vi "Serial_Terminal.vi"() -> ()   [LabVIEW 2009]
uses:
  <vilib>/Instr/_visa.llb/VISA Configure Serial Port (Instr).vi
panel:
  in  "baud rate (9600)":u32=38400
  in  "Send Style":u16(ring) items=["Slash Codes"=1, "HEX"=3, "ASCII"=0]
  in  "Send":bool
  in  "Input":string
  in  "Selection Style":u16(ring)=3 items=["Slash Codes"=1, "HEX"=3, "ASCII"=0]
  out "concatenated string 2":string
  in  "Display Style":u16(ring) items=["Slash Codes"=1, "HEX"=3, "ASCII"=0]
  in  "reset":bool
  in  "clear":bool
  in  "start/stop":bool=TRUE
  in  "VISA resource name":refnum<visa-resource-name>
  out "concatenated string":string
  in  "stop":bool
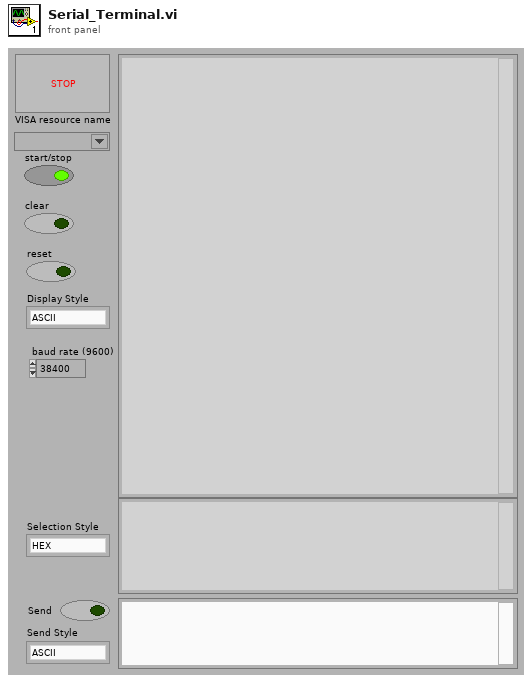
[diagram p1: front panel]
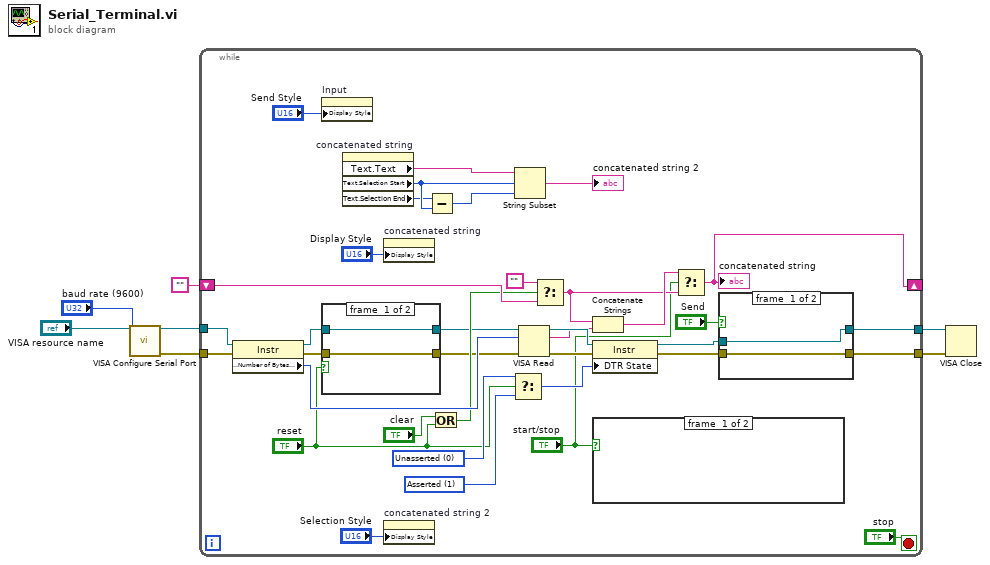
[diagram p0: block diagram]
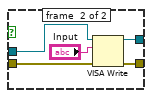
[diagram p2: hidden frame]
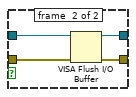
[diagram p3: hidden frame]
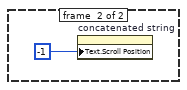
[diagram p4: hidden frame]
diagram:
  n1 = call-poly "VISA Configure Serial Port"("VISA resource name"="VISA resource name", "baud rate (9600)"="baud rate (9600)") -> ("VISA resource name out"=w5:refnum<visa-resource-name>, "error out"=w6:errorcluster)  [unwired: 12 in]
  n2 = while {
    shift-right: [w39] -> _
    shift-left: "" -> [w37]
    tunnel: w5 -> [w9]
    tunnel: w6 -> [w8]
    tunnel: [w11] -> w4
    tunnel: [w10] -> w3
    stop <- "stop" stop-if-true
    w34 = i16 1 items=["Unknown"=-1, "Unasserted"=0, "Asserted"=1] ("Serial Settings:Modem Line Settings:Line DTR State")
    w35 = i16 0 items=["Unknown"=-1, "Unasserted"=0, "Asserted"=1] ("Serial Settings:Modem Line Settings:Line DTR State")
    n3 = property class="Instr"(reference=w9, error in=w8) -> (reference out=w25:refnum<visa-resource-name>, error out=w24:errorcluster, "Serial Settings:Number of Bytes at Serial Port"=w42:u32)
    n4 = property on="Input" class="Str"("Display Style"="Send Style") -> ()  [unwired: 2 in, 2 out]
    n5 = case shown="False" "reset" {
      tunnel: w25 -> [w52 w56]
      tunnel: [w52 w55] -> w22
      tunnel: w24 -> [w51 w54]
      tunnel: [w51 w53] -> w23
      frame #0 {
      }
      frame #1 {
        n6 = VISA Flush I/O Buffer(VISA resource name=w56, error in (no error)=w54) -> (VISA resource name out=w55:refnum<visa-resource-name>, error out=w53:errorcluster)  [unwired: 1 in]
      }
    }
    n7 = property on="concatenated string" class="Str"() -> ("Text.Text"=w21:string, "Text.Selection Start"=w20:u32, "Text.Selection End"=w19:u32)  [unwired: 2 in, 2 out]
    n8 = property on="concatenated string" class="Str"("Display Style"="Display Style") -> ()  [unwired: 2 in, 2 out]
    n9 = property on="concatenated string 2" class="Str"("Display Style"="Selection Style") -> ()  [unwired: 2 in, 2 out]
    n10 = Subtract(x=w19, y=w20) -> (x-y=w18:u32)
    n11 = Or(x="clear", y="reset") -> (x .or. y?=w27:bool)
    n12 = Select(t=w35, s="reset", f=w34) -> (s? t:f=w33:i16)
    n13 = String Subset(string=w21, offset (0)=w20, length (rest)=w18) -> (substring=→"concatenated string 2":string)
    n14 = VISA Read(VISA resource name=w22, byte count=w42, error in (no error)=w23) -> (VISA resource name out=w41:refnum<visa-resource-name>, read buffer=w31:string, error out=w40:errorcluster)  [unwired: 1 out]
    n15 = Select(t="", s=w27, f=w37) -> (s? t:f=w32:string)
    n16 = Concatenate Strings(w32, w31) -> (w38:string)
    n17 = property class="Instr"(reference=w41, error in=w40, "DTR State"=w33) -> (reference out=w13:refnum<visa-resource-name>, error out=w12:errorcluster)
    n18 = case shown="True" "start/stop" {
      frame #0 {
      }
      frame #1 {
        n19 = property on="concatenated string" class="Str"("Text.Scroll Position"=-1) -> ()  [unwired: 2 in, 2 out]
      }
    }
    n20 = Select(t=w38, s="start/stop", f=w32) -> (s? t:f=w39:string)
    "concatenated string" <- w39
    n21 = case shown="True" "Send" {
      tunnel: w13 -> [w45 w47]
      tunnel: w12 -> [w44 w48]
      tunnel: [w45 w50] -> w11
      tunnel: [w44 w49] -> w10
      frame #0 {
      }
      frame #1 {
        n22 = VISA Write(VISA resource name=w47, write buffer="Input", error in (no error)=w48) -> (VISA resource name out=w50:refnum<visa-resource-name>, error out=w49:errorcluster)  [unwired: 1 out]
      }
    }
  }
  n23 = VISA Close(VISA resource name=w4, error in (no error)=w3) -> ()  [unwired: 1 out]
